vi "5.11-TCP Data Client.vi"() -> ()   [LabVIEW 2011]
doc: "Displays data sent via TCP from Data Server.vi. Once a TCP connection is open, the VI reads 4 bytes to determine the amount of data being sent. It then reads and charts that many bytes. If an error occurs or the stop button is pressed, it sends a \"Q\" to the Data Sender to notify it to quit.\n\n<B>Note:</B> Requires the Data Server.vi located in the same library as this VI."
uses:
  5.0-Global.vi
panel:
  in  "Address":string="10.10.10.2"
  in  "Port":u16=33483 min=1025 step=1
  # "Instructions:\n1. Open the Data Server.vi located in the same library.\n2. Follow the instructions on it's front panel.\n\nNote: This VI is built to work with the Data Server.vi."
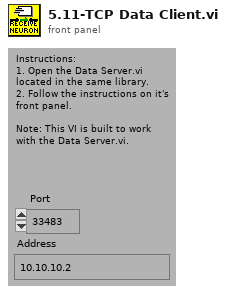
[diagram p1: front panel]
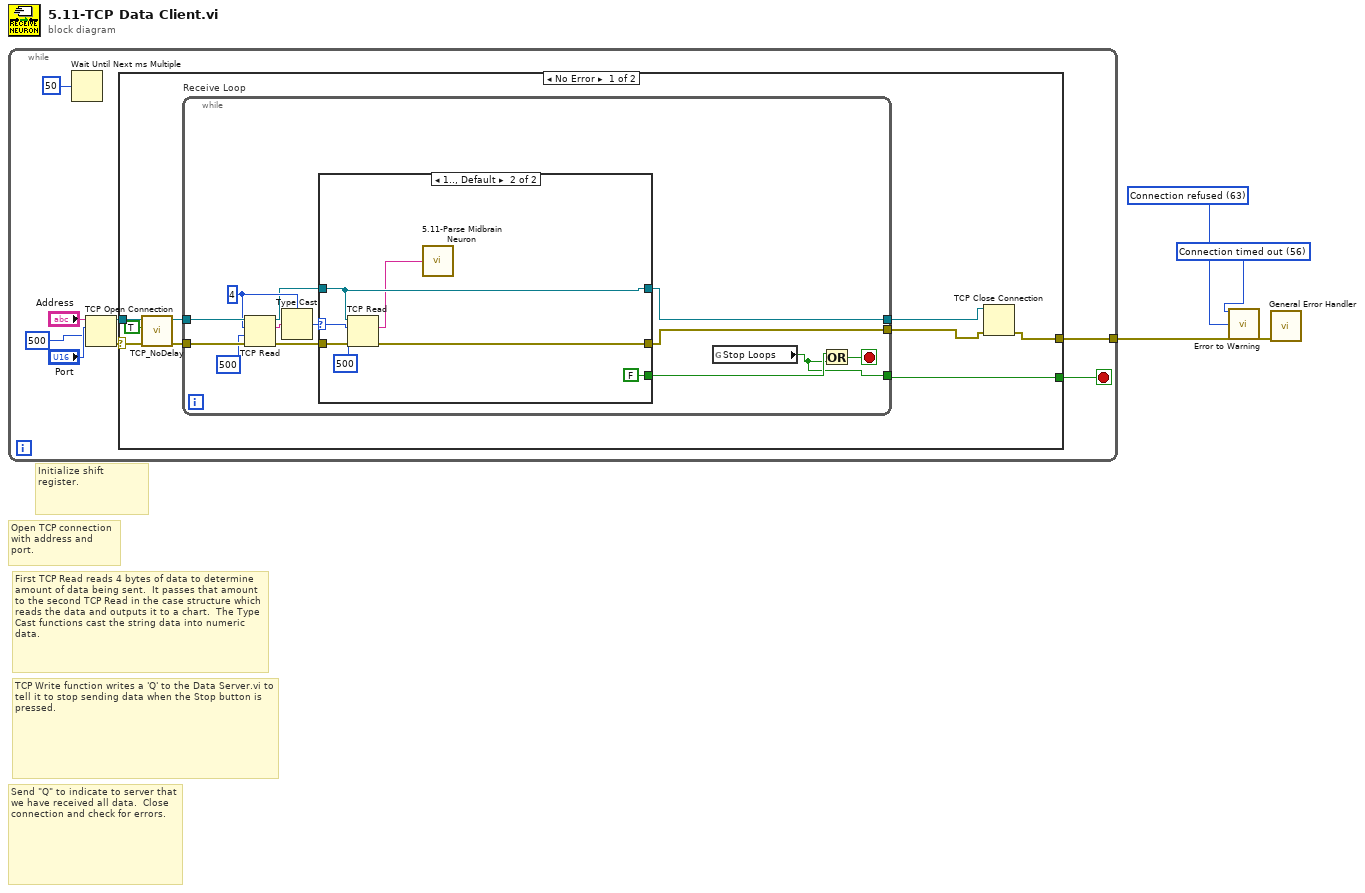
[diagram p0: block diagram]
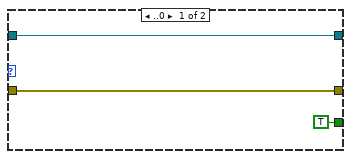
[diagram p2: hidden frame]
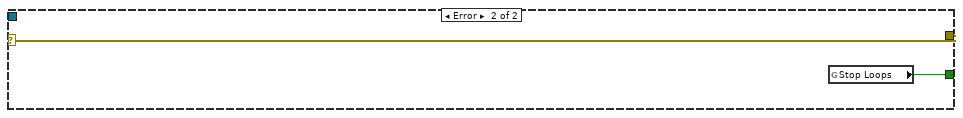
[diagram p3: hidden frame]
diagram:
  w1 = 63 items=["No Error", "Argument Error", "Memory Full", "Out of Zone", "End of File", "File Already Open", "Generic File IO Error", "File Not Found", "File Permission Error", "Disk Full", "Duplicate Path", "Too Many Files Open", "Not Enabled", "Resource File Not Found", "Cannot Add Resource", "Resource Not Found", "Image Not Found", "Image Memory Error", "Pen Does Not Exist", "Config Bad Type", "Config Token Not Found", "Config Parse Error", "Config Memory Error", "Bad External Code Format", "Bad External Code Offset", "External Code Not Present", "Null Window", "Destroy Window Mixup", "Null Menu", "Print Aborted", "Bad Print Record", "Print Driver Error", "Windows Error During Print", "Memory Error During Print", "Print Dialog Error", "Generic Print Error", "Invalid Device Refnum", "Device Not Found", "Device Parameter Error", "Device Unit Error", "Can't Open Device", "Device Call Aborted", "Generic Error", "Cancelled By User", "Object ID Too Low", "Object ID Too High", "Object Not In Heap", "Unknown Heap", "Bad DefProc ID", "DefProc Not In Table", "Message Out Of Range", "Null Method", "Unknown Message", "Manager Call Not Supported", "Bad address", "Connection In progress", "Connection timed out", "Connection is already in progress", "Network attribute not supported", "Network error", "Address in use", "System out of memory", "Connection aborted", "Connection refused", "Connection is not connected", "Connection is already connected", "Connection closed", "Initialize error (interapplication manager)", "Bad occurrence", "Wait on unbound occurrence handler", "Occurrence queue overflow", "Bad path", "Semaphore not signaled", "Unrecognized type (interapplication manager)"] ("3rd Error to Convert")
  w4 = 56 items=["No Error", "Argument Error", "Memory Full", "Out of Zone", "End of File", "File Already Open", "Generic File IO Error", "File Not Found", "File Permission Error", "Disk Full", "Duplicate Path", "Too Many Files Open", "Not Enabled", "Resource File Not Found", "Cannot Add Resource", "Resource Not Found", "Image Not Found", "Image Memory Error", "Pen Does Not Exist", "Config Bad Type", "Config Token Not Found", "Config Parse Error", "Config Memory Error", "Bad External Code Format", "Bad External Code Offset", "External Code Not Present", "Null Window", "Destroy Window Mixup", "Null Menu", "Print Aborted", "Bad Print Record", "Print Driver Error", "Windows Error During Print", "Memory Error During Print", "Print Dialog Error", "Generic Print Error", "Invalid Device Refnum", "Device Not Found", "Device Parameter Error", "Device Unit Error", "Can't Open Device", "Device Call Aborted", "Generic Error", "Cancelled By User", "Object ID Too Low", "Object ID Too High", "Object Not In Heap", "Unknown Heap", "Bad DefProc ID", "DefProc Not In Table", "Message Out Of Range", "Null Method", "Unknown Message", "Manager Call Not Supported", "Bad address", "Connection In progress", "Connection timed out", "Connection is already in progress", "Network attribute not supported", "Network error", "Address in use", "System out of memory", "Connection aborted", "Connection refused", "Connection is not connected", "Connection is already connected", "Connection closed", "Initialize error (interapplication manager)", "Bad occurrence", "Wait on unbound occurrence handler", "Occurrence queue overflow", "Bad path", "Semaphore not signaled", "Unrecognized type (interapplication manager)"] ("1st Error to Convert")
  # "Initialize shift register."
  # "Send \"Q\" to indicate to server that we have received all data.  Close connection and check for errors."
  # "TCP Write function writes a 'Q' to the Data Server.vi to tell it to stop sending data when the Stop button is pressed."
  # "First TCP Read reads 4 bytes of data to determine amount of data being sent.  It passes that amount to the second TCP Read in the case structure which reads the data and outputs it to a chart.  The Type Cast functions cast the string data into numeric data."
  # "Open TCP connection with address and port."
  n1 = while {
    tunnel: [w6] -> w2
    stop <- w7 stop-if-true
    n2 = Wait Until Next ms Multiple(millisecond multiple=u32 50) -> ()  [unwired: 1 out]
    n3 = TCP Open Connection(address="Address", remote port or service name="Port", timeout ms (60000)=500) -> (connection ID=w10:refnum<k5>, error out=w9:errorcluster)  [unwired: 1 in, 1 out]
    n4 = case shown="No Error" w9 {
      selector: w9 -> [w18 w45]
      tunnel: w10 -> [w20 _]
      tunnel: [w21 w46] -> w7
      tunnel: [w13 w45] -> w6
      frame No Error {
        n5 = call "TCP_NoDelay.vi"("error in (no error)"=w18, "TCP_NODELAY (true)"=TRUE, "connID"=w20) -> ("error out"=w17:errorcluster, "connID 2"=w19:refnum<k5>)  [unwired: 3 in]
        n6 = while "Receive Loop" {
          tunnel: w17 -> [w32]
          tunnel: w19 -> [w33]
          tunnel: [w22] -> w21
          tunnel: [w26] -> w15
          tunnel: [w25] -> w14
          stop <- w24 stop-if-true
          w31 = 4
          n7 = TCP Read(connection ID=w33, bytes to read=w31, error in (no error)=w32, 9:500 ("timeout ms (25000)")) -> (connection ID out=w28:refnum<k5>, data out=w34:string, error out=w29:errorcluster)  [unwired: 1 out]
          n8 = Type Cast(type=w31, x=w34) -> (*(type *) &x=w30:i32)
          n9 = case shown="1.., Default" w30 {
            selector: w30 -> [_ w43]
            tunnel: w29 -> [w35 w44]
            tunnel: w28 -> [w37 w41]
            tunnel: [w37 w41] -> w26
            tunnel: [TRUE FALSE] -> w27
            tunnel: [w35 w38] -> w25
            frame ..0 {
            }
            frame 1.., Default {
              n10 = TCP Read(connection ID=w41, bytes to read=w43, error in (no error)=w44, 9:500 ("timeout ms (25000)")) -> (data out=w39:string, error out=w38:errorcluster)  [unwired: 2 out]
              n11 = call "5.11-Parse Midbrain Neuron.vi"("data out"=w39) -> ()
            }
          }
          n12 = global read "5.0-Global.vi" "Stop Loops"() -> (w22:bool)
          n13 = Or(x=w27, y=w22) -> (x .or. y?=w24:bool)
        }
        n14 = TCP Close Connection(connection ID=w15, error in (no error)=w14) -> (error out=w13:errorcluster)  [unwired: 2 out]
      }
      frame Error {
        n15 = global read "5.0-Global.vi" "Stop Loops"() -> (w46:bool)
      }
    }
  }
  n16 = call <vilib>:"Error to Warning.vi"("1st Error to Convert"=w4, "3rd Error to Convert"=w1, "error in"=w2) -> ("warning out"=w3:errorcluster)  [unwired: 12 in]
  n17 = call <vilib>:"General Error Handler.vi"("error in (no error)"=w3) -> ()  [unwired: 2 in, 13 out]
